vi "niScope EX Configured Acquisition.vi"() -> ()   [LabVIEW 2021]
doc: "Recommended Input Signal: 100 kHz, 4 Vpp, sine wave\n\nDevices Supported: Refer to NI Example Finder\n\nThis example configures all the oscilloscope's vertical, horizontal, and triggering properties before every acquisition. It allows you to experiment with numerous configurations, including acquisition types and triggering modes, since it supports nearly the entire functionality of NI-SCOPE. However, it is may be more instructive to consult other examples about specific topics such as FlexRes, Random Interleaved Sampling, and Multi-Record to learn more about these features.\n\nMany parameters are included an the front panel of this example. Notice that the \"min sample rate\" is next to the \"actual sample rate,\" and similarly the \"min record length\" is near the \"actual record length.\" The \"min\" values are specified with the Configure Horizontal Timing VI. NI-SCOPE maintains a constant time per record for each acquisition. So when you specify a min sample rate and a min record length, this determines the amount of time the acquisition should take:\n\n time per record = min record length / min sampling rate. \n\nHowever, oscilloscopes support only a certain number of defined sampling rates, so if the value chosen is not a valid rate, it is rounded to the next higher rate, called the actual sample rate. The actual record length is then calculated in order to maintain the time per record. Both of these values are returned in this example so you can investigate the effects of parameter rounding with your oscilloscope. For more information about parameter coercions, see the NI High Speed Digitizers Help.\n\nThe enforce realtime property allows this example to use Random Interleaved Sampling. See the Random Interleaved Sampling example for more details.\n\nKeep in mind that not all digitizers/oscilloscopes support all the features in this example. The NI High Speed Digitizers Help includes a table of supported features for each device."
uses:
  Controls/Clusts/Scope_Cfg_Clust.ctl
  Controls/Clusts/Resource_Cfg_Clust.ctl
  Controls/Clusts/Vertical_Cfg_Clust.ctl
  Controls/Clusts/Horizontal_Cfg_Clust.ctl
  Controls/Clusts/Trig_Cfg_Clust.ctl
  Controls/Enums/Trig_Type_Enum.ctl
  Controls/Clusts/Trig_Edge_Cfg_Clust.ctl
  Controls/Clusts/Trig_Dig_Cfg_Clust.ctl
  Controls/Enums/Scope_Loop_Enum.ctl
  <instrlib>/niScope/Utility/niScope Get Channel Name From String.vi
  <instrlib>/niScope/Configure/Trigger/niScope Configure Trigger Immediate.vi
  <instrlib>/niScope/Configure/Trigger/niScope Configure Trigger Edge.vi
  <instrlib>/niScope/Configure/Trigger/niScope Configure Trigger Digital.vi
  <instrlib>/niScope/Acquire/Fetch/niScope Multi Fetch Cluster.vi
panel:
  out "Index":i32
  in  "Scope":T1={"instrument handle"="", "TaskRef"="", "channel name"="", "Resource"={"Resource Name"="Dev1", "Channel Name"="0", "Timeout (s)"=5.0}, "Vert"={"Vertical Range"=5.0, "Vertical Offset"=0.0, "Probe Attenuation"=1.0, "Vertical Coupling"=1}, "Hor"={"Maximum Input Frequency"=0.0, "Min Sample Rate"=10000000.0, "Min Record Length"=1000}, "Trig"={"Trigger Modifier"=2, "Trigger Delay"=0.0, "Reference Position"=50.0, "TrigType"=enum."Immediate", "Edge"={"Coupling"=1, "Trigger Slope"=0, "Trigger Source"="0", "Trigger Level"=0.0}, "Dig"={"Trigger Source"="VAL_PFI_1", "Trigger Slope"=0}}} {"Trig"."Dig"."Trigger Slope" items=["Positive", "Negative"]; "Trig"."Edge"."Trigger Level" format="%.2f"; "Trig"."Edge"."Trigger Slope" items=["Positive", "Negative"]; "Trig"."Edge"."Coupling" items=["AC"=0, "DC"=1, "HF Reject"=3, "LF Reject"=4, "AC Plus HF Reject"=1001]; "Trig"."Reference Position" format="%.1f"; "Trig"."Trigger Delay" format="%#.4p"; "Trig"."Trigger Modifier" items=["None"=1, "Auto Trigger"=2]; "Hor"."Min Sample Rate" step=1000000.0 format="%#.2p"; "Hor"."Maximum Input Frequency" format="%.2f"; "Vert"."Vertical Coupling" items=["AC", "DC", "Ground"]; "Vert"."Probe Attenuation" format="%.1f"; "Vert"."Vertical Offset" format="%.2p"; "Vert"."Vertical Range" format="%.2f"; "Resource"."Timeout (s)" format="%.2f"}
  out "Auto Triggered":bool
  out "Actual Sample Rate":dbl=10000000.0 format="%#.2p"
  out "Actual Record Length":i32=1000
  out "Waveform(s)":T9(graph)
  # "Overview: Demonstrates how to configure vertical, horizontal, and triggering properties and allows you to experiment with numerous configurations, including acquisition types and triggering mode.\nRequirements: NI-SCOPE\nInstructions: \n1. Configure desired acquisition settings.\n2. Run the VI.\n3. Click Stop to stop the VI."
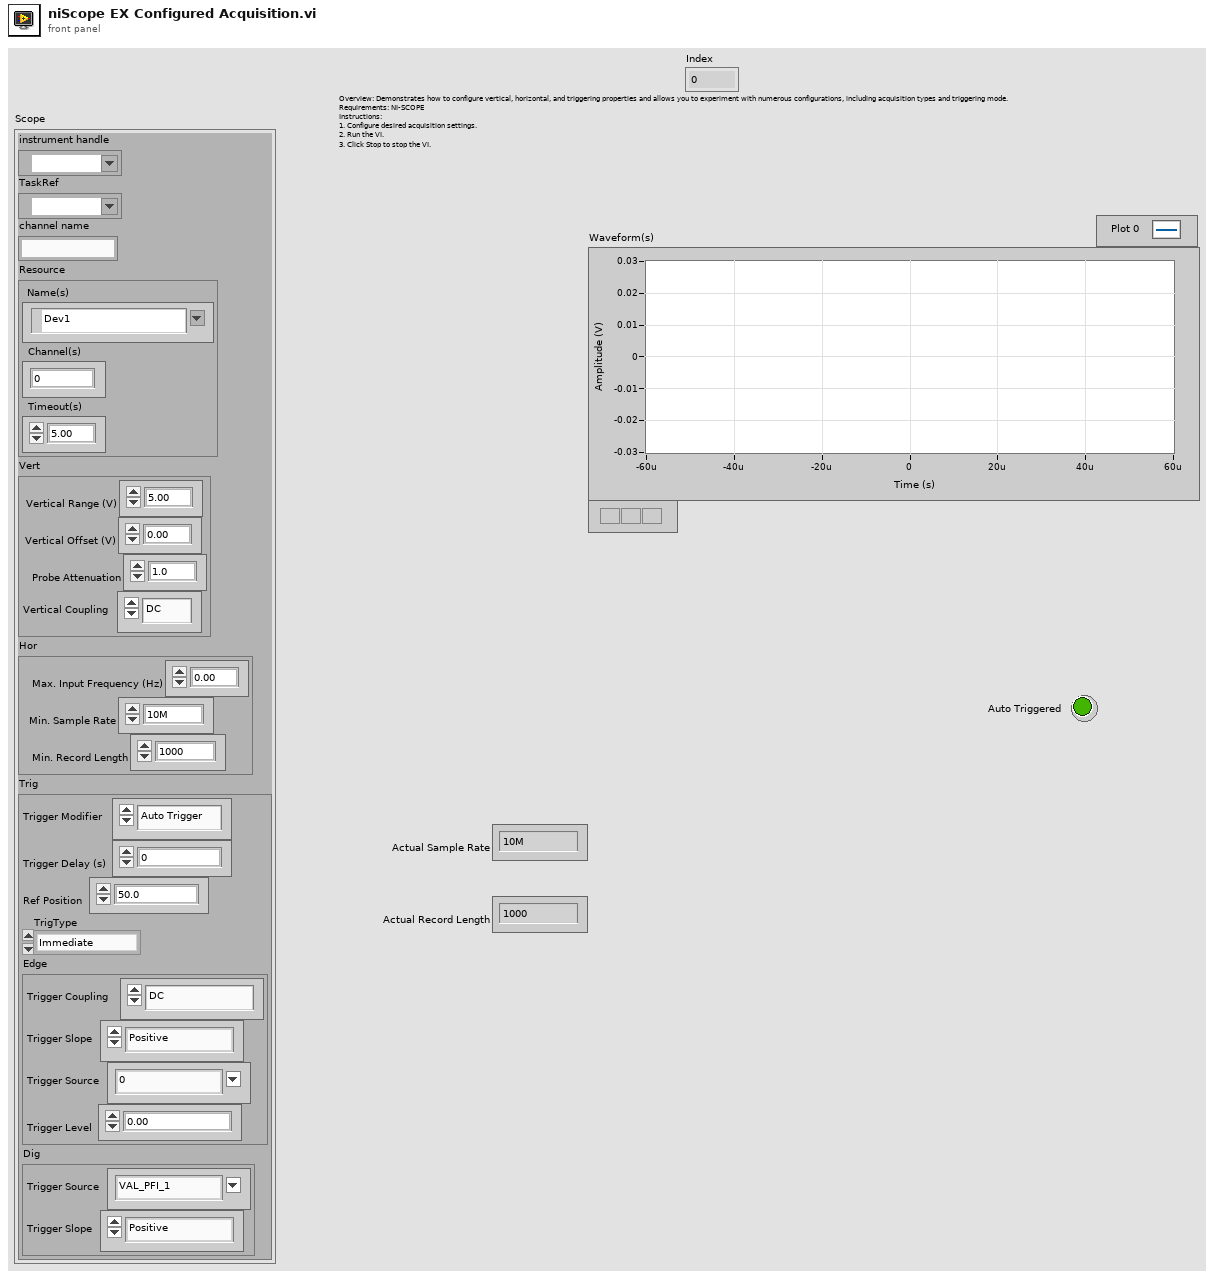
[diagram p1: front panel]
types:
  T1 = typedef "Scope_Cfg_Clust.ctl" = cluster{"instrument handle":refnum<k15>, "TaskRef":refnum<k15>, "channel name":string, "Resource":T2, "Vert":T3, "Hor":T4, "Trig":T5}
  T2 = typedef "Resource_Cfg_Clust.ctl" = cluster{"Resource Name":refnum<k15>, "Channel Name":string, "Timeout (s)":dbl}
  T3 = typedef "Vertical_Cfg_Clust.ctl" = cluster{"Vertical Range":dbl, "Vertical Offset":dbl, "Probe Attenuation":dbl, "Vertical Coupling":i32}
  T4 = typedef "Horizontal_Cfg_Clust.ctl" = cluster{"Maximum Input Frequency":dbl, "Min Sample Rate":dbl, "Min Record Length":i32}
  T5 = typedef "Trig_Cfg_Clust.ctl" = cluster{"Trigger Modifier":i32, "Trigger Delay":dbl, "Reference Position":dbl, "TrigType":T6, "Edge":T7, "Dig":T8}
  T6 = typedef "Trig_Type_Enum.ctl" = enum16{"Immediate", "Edge", "Digital"}
  T7 = typedef "Trig_Edge_Cfg_Clust.ctl" = cluster{"Coupling":u16, "Trigger Slope":i32, "Trigger Source":string, "Trigger Level":dbl}
  T8 = typedef "Trig_Dig_Cfg_Clust.ctl" = cluster{"Trigger Source":string, "Trigger Slope":i32}
  T9 = cluster{"relativeInitialX":dbl, "xIncrement":dbl, "wfm":dbl[]}[]
  T10 = typedef "Scope_Loop_Enum.ctl" = enum16{"Init", "Cfg", "Read", "Stop", "Close"}
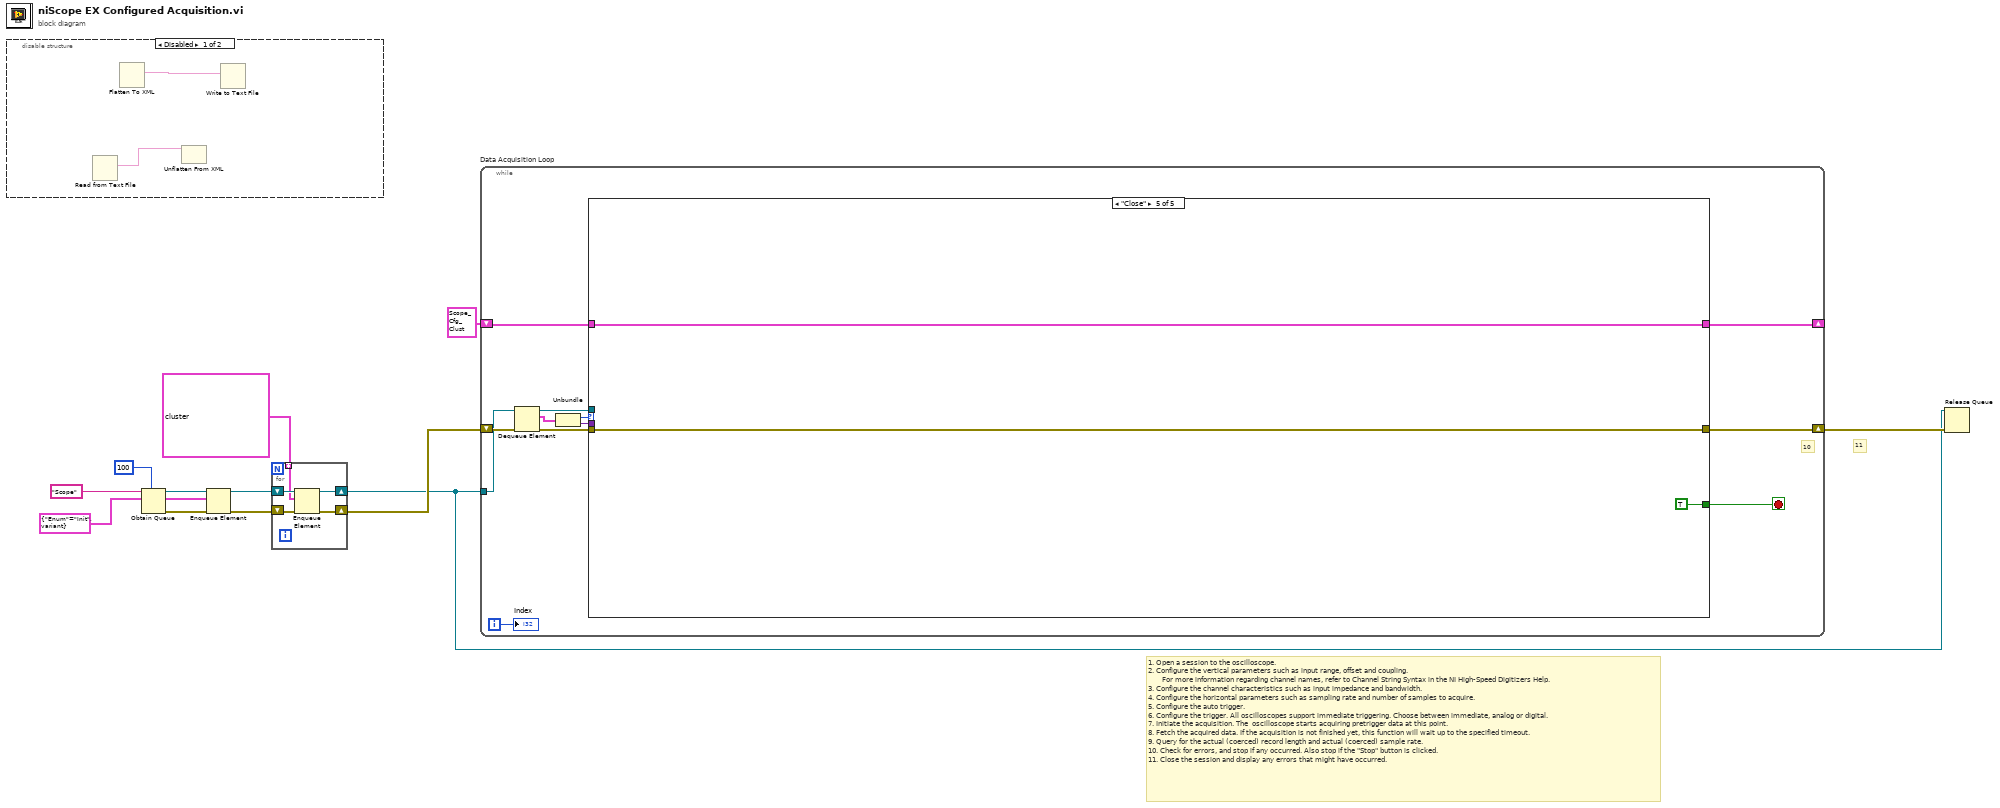
[diagram p0: block diagram]
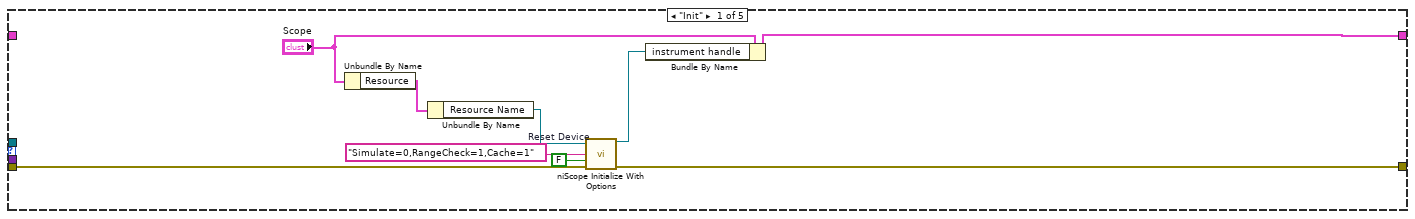
[diagram p3: hidden frame]
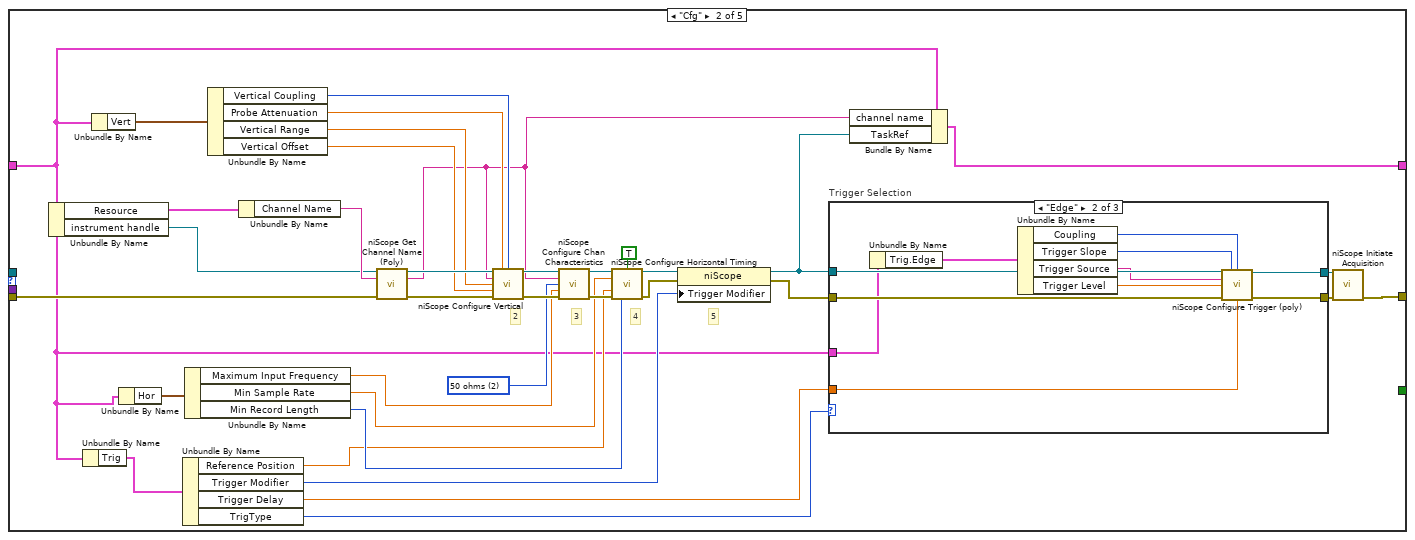
[diagram p4: hidden frame]
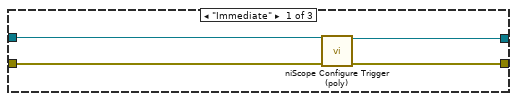
[diagram p5: hidden frame]
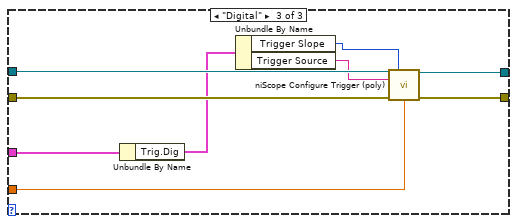
[diagram p6: hidden frame]
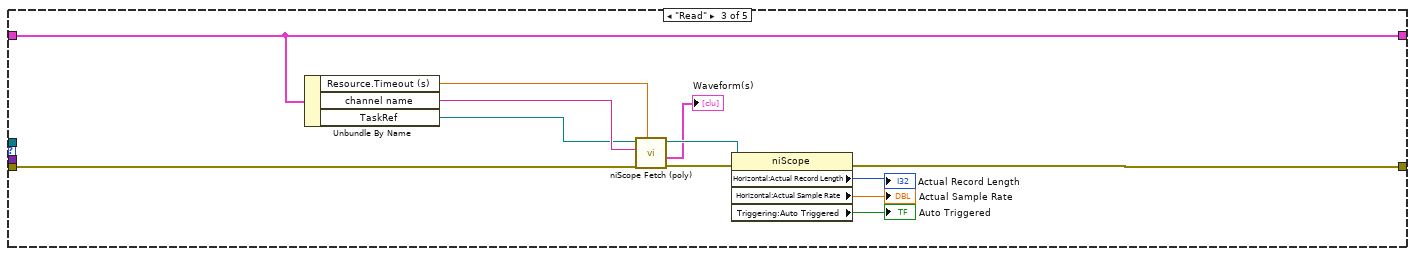
[diagram p7: hidden frame]
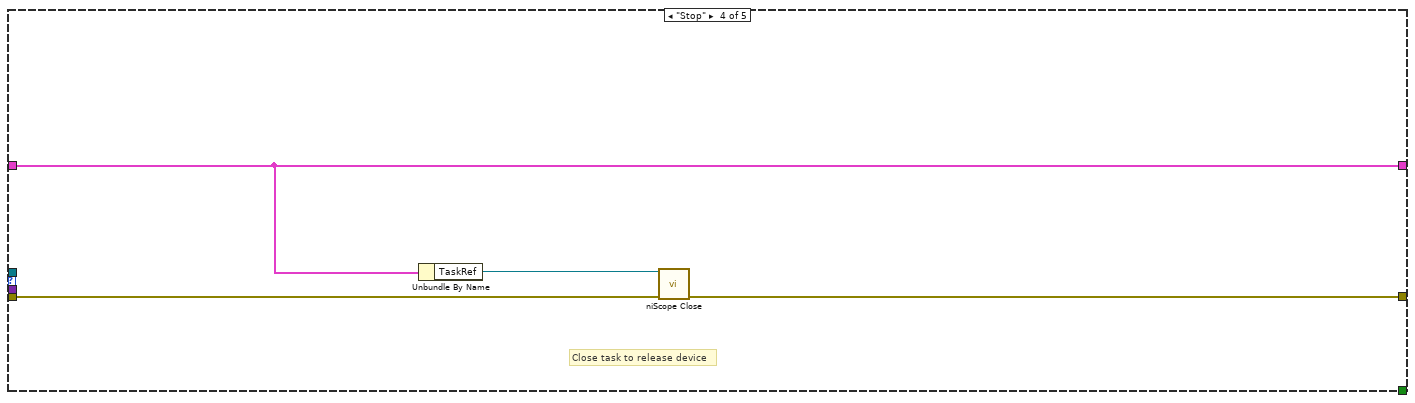
[diagram p8: hidden frame]
diagram:
  w9 = cluster{"Enum":T10, variant} {"Enum"=enum."Init", variant}
  # "1. Open a session to the oscilloscope.\n2. Configure the vertical parameters such as input range, offset and coupling.\n       For more information regarding channel names, refer to Channel String Syntax in the NI High-Speed Digitizers Help.\n3. Configure the channel characteristics such as input impedance and bandwidth.\n4. Configure the horizontal parameters such as sampling rate and number of samples to acquire.\n5. Configure the auto trigger.\n6. Configure the trigger. All oscilloscopes support immediate triggering. Choose between immediate, analog or digital.\n7. Initiate the acquisition. The  oscilloscope starts acquiring pretrigger data at this point.\n8. Fetch the acquired data. If the acquisition is not finished yet, this function will wait up to the specified timeout.\n9. Query for the actual (coerced) record length and actual (coerced) sample rate.\n10. Check for errors, and stop if any occurred. Also stop if the \"Stop\" button is clicked.\n11. Close the session and display any errors that might have occurred."
  # "11"
  n1 = disable-structure shown="Disabled" {
    frame Disabled {
      n2 = Read from Text File() -> (text=w13:string)  [unwired: 4 in, 3 out]
      n3 = Flatten To XML() -> (2:w14:string)  [unwired: 1 in]
      n4 = Unflatten From XML(xml string=w13) -> ()  [unwired: 2 in, 2 out]
      n5 = Write to Text File(text=w14) -> ()  [unwired: 3 in, 3 out]
    }
    frame Enabled {
    }
  }
  n6 = Obtain Queue(max queue size (-1, unlimited)=100, name (unnamed)="Scope", element data type=w9) -> (queue out=w8:refnum<queue>, error out=w10:errorcluster)  [unwired: 2 in, 1 out]
  n7 = Enqueue Element(queue=w8, element=w9, error in (no error)=w10) -> (queue out=w6:refnum<queue>, error out=w5:errorcluster)  [unwired: 1 in, 1 out]
  n8 = for {
    tunnel: cluster{"Enum":T10, variant}[] [{"Enum"=enum."Cfg", variant}, {"Enum"=enum."Read", variant}, {"Enum"=enum."Stop", variant}, {"Enum"=enum."Close", variant}] -> [w15] mode=indexing
    shift-right: [w19] -> w1
    shift-left: w6 -> [w18]
    shift-right: [w16] -> w4
    shift-left: w5 -> [w17]
    n9 = Enqueue Element(queue=w18, element=w15, error in (no error)=w17) -> (queue out=w19:refnum<queue>, error out=w16:errorcluster)  [unwired: 1 in, 1 out]
  }
  n10 = while "Data Acquisition Loop" {
    shift-right: [w23] -> w2
    shift-left: w4 -> [w29]
    shift-right: [w22] -> _
    shift-left: T1 {"instrument handle"="", "TaskRef"="", "channel name"="", "Resource"={"Resource Name"="Dev1", "Channel Name"="0", "Timeout (s)"=5.0}, "Vert"={"Vertical Range"=5.0, "Vertical Offset"=0.0, "Probe Attenuation"=1.0, "Vertical Coupling"=1}, "Hor"={"Maximum Input Frequency"=0.0, "Min Sample Rate"=10000000.0, "Min Record Length"=1000}, "Trig"={"Trigger Modifier"=2, "Trigger Delay"=0.0, "Reference Position"=50.0, "TrigType"=enum."Immediate", "Edge"={"Coupling"=1, "Trigger Slope"=0, "Trigger Source"="0", "Trigger Level"=0.0}, "Dig"={"Trigger Source"="VAL_PFI_1", "Trigger Slope"=0}}} ("Scope") -> [w30]
    tunnel: w1 -> [w28]
    i -> [w20]
    stop <- w21 stop-if-true
    # "10"
    n11 = Dequeue Element(queue=w28, error in (no error)=w29) -> (queue out=w27:refnum<queue>, element=w26:cluster{"Enum":T10, variant})  [unwired: 1 in, 2 out]
    n12 = Unbundle(w26) -> ("Enum"=w25:T10, w24:variant)
    n13 = case shown="\"Close\"" w25 {
      tunnel: [w32 w69 w100 w114 w117] -> w23
      tunnel: w29 -> [w33 w61 w101 w115 w117]
      tunnel: w30 -> [_ w43 w103 w112 w116]
      tunnel: w27 -> [_ _ _ _ _]
      tunnel: w24 -> [_ _ _ _ _]
      tunnel: [w31 w42 w103 w112 w116] -> w22
      tunnel: [_ _ _ _ TRUE ("Stop")] -> w21
      frame "Init" {
        w34 = FALSE  # Reset Device
        n14 = Unbundle By Name("Scope") -> ("Resource"=w37:T2)
        n15 = Unbundle By Name(w37) -> ("Resource Name"=w36:refnum<k15>)
        n16 = call <instrlib>:"niScope Initialize With Options.vi"("resource name"=w36, "option string"="Simulate=0,RangeCheck=1,Cache=1", "reset device"=w34, "error in"=w33) -> ("instrument handle"=w39:refnum<k15>, "error out"=w32:errorcluster)  [unwired: 10 in]
        n17 = Bundle By Name(cluster="Scope", "instrument handle"=w39) -> (w31:T1)
      }
      frame "Cfg" {
        w71 = u32 2 items=["1 mega ohm"=0, "50 ohms"=2] ("Input Impedance")
        # "5"
        # "2"
        # "3"
        # "4"
        n18 = Unbundle By Name(w43) -> ("Resource"=w47:T2, "instrument handle"=w44:refnum<k15>)
        n19 = Unbundle By Name(w43) -> ("Trig"=w46:T5)
        n20 = Unbundle By Name(w43) -> ("Vert"=w48:T3)
        n21 = Unbundle By Name(w43) -> ("Hor"=w45:T4)
        n22 = Unbundle By Name(w46) -> ("Reference Position"=w52:dbl, "Trigger Modifier"=w51:i32, "Trigger Delay"=w50:dbl, "TrigType"=w49:T6)
        n23 = Unbundle By Name(w45) -> ("Maximum Input Frequency"=w55:dbl, "Min Sample Rate"=w54:dbl, "Min Record Length"=w53:i32)
        n24 = Unbundle By Name(w48) -> ("Vertical Coupling"=w59:i32, "Probe Attenuation"=w58:dbl, "Vertical Range"=w57:dbl, "Vertical Offset"=w56:dbl)
        n25 = Unbundle By Name(w47) -> ("Channel Name"=w60:string)
        n26 = call-poly <instrlib>:"niScope Get Channel Name (Poly).vi"("instrument handle"=w44, "index"=w60, "error in"=w61) -> ("instrument handle out"=w63:refnum<k15>, "channel name"=w41:string, "error out"=w62:errorcluster)  [unwired: 10 in]
        n27 = call <instrlib>:"niScope Configure Vertical.vi"("instrument handle"=w63, "probe attenuation"=w58, "vertical coupling"=w59, "channels"=w41, "vertical range"=w57, "vertical offset"=w56, "error in"=w62) -> ("instrument handle out"=w75:refnum<k15>, "error out"=w74:errorcluster)  [unwired: 7 in]
        n28 = call <instrlib>:"niScope Configure Chan Characteristics.vi"("instrument handle"=w75, "channels"=w41, "input impedance"=w71, "maximum input frequency"=w55, "error in"=w74) -> ("instrument handle out"=w72:refnum<k15>, "error out"=w73:errorcluster)  [unwired: 9 in]
        n29 = call <instrlib>:"niScope Configure Horizontal Timing.vi"("instrument handle"=w72, "enforce realtime"=TRUE ("Enforce Realtime"), "min sample rate"=w54, "reference position"=w52, "error in"=w73, "min record length"=w53) -> ("instrument handle out"=w67:refnum<k15>, "error out"=w66:errorcluster)  [unwired: 8 in]
        n30 = property on="Property Node" class="niScope"(reference=w67, error in=w66, "Trigger Modifier"=w51) -> (reference out=w40:refnum<k15>, error out=w65:errorcluster)
        n31 = case "Trigger Selection" shown="\"Edge\"" w49 {
          tunnel: w65 -> [w79 w90 w99]
          tunnel: [w76 w86 w95] -> w68
          tunnel: w40 -> [w78 w89 w98]
          tunnel: [w77 w87 w96] -> w70
          tunnel: w50 -> [_ w88 w97]
          tunnel: w43 -> [_ w80 w92]
          frame "Immediate" {
            n32 = call-poly <instrlib>:"niScope Configure Trigger (poly).vi"("instrument handle"=w78, "error in"=w79) -> ("instrument handle out"=w77:refnum<k15>, "error out"=w76:errorcluster)  [unwired: 12 in]
          }
          frame "Edge" {
            n33 = Unbundle By Name(w80) -> ("Trig.Edge"=w81:T7)
            n34 = Unbundle By Name(w81) -> ("Coupling"=w85:u16, "Trigger Slope"=w84:i32, "Trigger Source"=w83:string, "Trigger Level"=w82:dbl)
            n35 = call-poly <instrlib>:"niScope Configure Trigger (poly).vi"("instrument handle"=w89, "trigger slope"=w84, "trigger coupling"=w85, "trigger source"=w83, "trigger level"=w82, "error in"=w90, "trigger delay"=w88) -> ("instrument handle out"=w87:refnum<k15>, "error out"=w86:errorcluster)  [unwired: 7 in]
          }
          frame "Digital" {
            n36 = Unbundle By Name(w92) -> ("Trig.Dig"=w91:T8)
            n37 = Unbundle By Name(w91) -> ("Trigger Slope"=w93:i32, "Trigger Source"=w94:string)
            n38 = call-poly <instrlib>:"niScope Configure Trigger (poly).vi"("instrument handle"=w98, "trigger slope"=w93, "trigger source"=w94, "error in"=w99, "trigger delay"=w97) -> ("instrument handle out"=w96:refnum<k15>, "error out"=w95:errorcluster)  [unwired: 9 in]
          }
        }
        n39 = Bundle By Name(cluster=w43, "channel name"=w41, "TaskRef"=w40) -> (w42:T1)
        n40 = call <instrlib>:"niScope Initiate Acquisition.vi"("instrument handle"=w70, "error in"=w68) -> ("error out"=w69:errorcluster)  [unwired: 12 in, 1 out]
      }
      frame "Read" {
        n41 = Unbundle By Name(w103) -> ("Resource.Timeout (s)"=w110:dbl, "channel name"=w111:string, "TaskRef"=w102:refnum<k15>)
        n42 = call-poly <instrlib>:"niScope Fetch (poly).vi"("timeout"=w110, "error in"=w101, "channels"=w111, "instrument handle"=w102) -> ("error out"=w106:errorcluster, "waveform"=→"Waveform(s)":T9, "instrument handle out"=w105:refnum<k15>)  [unwired: 4 in, 1 out]
        n43 = property class="niScope"(reference=w105, error in=w106) -> (error out=w100:errorcluster, "Horizontal:Actual Record Length"=→"Actual Record Length":i32, "Horizontal:Actual Sample Rate"=→"Actual Sample Rate":dbl, "Triggering:Auto Triggered"=→"Auto Triggered":bool)  [unwired: 1 out]
      }
      frame "Stop" {
        # "Close task to release device"
        n44 = Unbundle By Name(w112) -> ("TaskRef"=w113:refnum<k15>)
        n45 = call <instrlib>:"niScope Close.vi"("instrument handle"=w113, "error in"=w115) -> ("error out"=w114:errorcluster)  [unwired: 13 in]
      }
      frame "Close" {
      }
    }
    "Index" <- w20
  }
  n46 = Release Queue(queue=w1, error in (no error)=w2) -> ()  [unwired: 1 in, 3 out]
